vi "setStages.vi"(8 "error in (no error)":errorcluster, 10 "Stage":string, 11 "RfRamp.lvclass in":refnum<class "RfRamp.lvclass">) -> (0 "error out":errorcluster, 3 "RfRamp.lvclass out":refnum<class "RfRamp.lvclass">)   [LabVIEW 2011, in "Tools.lvlib" / "Scripting.lvlib" / "RfRamp.lvclass"]
uses:
  RfRamp.lvclass
  Rf Event/rf.lvclass
  RfRamp.lvclass/RfRamp.ctl
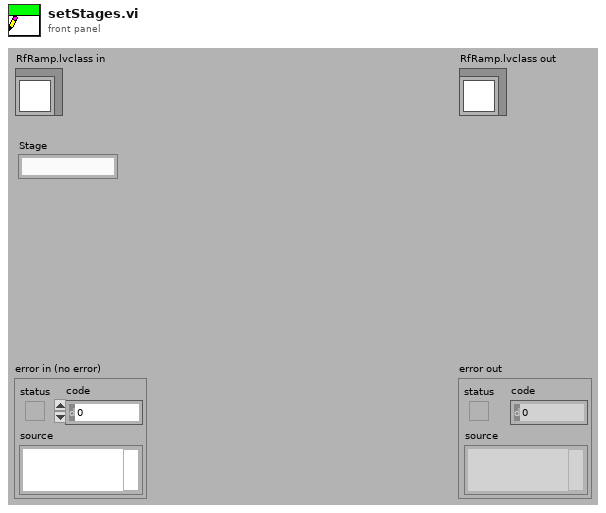
[diagram p1: front panel]
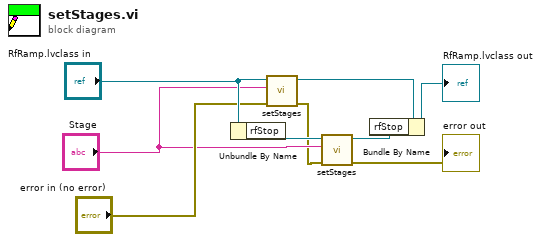
[diagram p0: block diagram]
diagram:
  n1 = Unbundle By Name("RfRamp.lvclass in") -> ("rfStop"=w3:refnum<class "rf.lvclass">)
  n2 = call-parent "setStages.vi"("error in (no error)"="error in (no error)", "Stage"="Stage", "ScriptEvent.lvclass in"="RfRamp.lvclass in") -> ("error out"=w1:errorcluster, "ScriptEvent.lvclass out"=w9:refnum<class "RfRamp.lvclass">)  [unwired: 7 in]
  n3 = call-dynamic "setStages.vi"("error in (no error)"=w1, "Stage"="Stage", "ScriptEvent.lvclass in"=w3) -> ("error out"=→"error out":errorcluster, "ScriptEvent.lvclass out"=w4:refnum<class "rf.lvclass">)  [unwired: 7 in]
  n4 = Bundle By Name(cluster=w9, "rfStop"=w4) -> (→"RfRamp.lvclass out":refnum<class "RfRamp.lvclass">)
